vi "calculate phase shift.vi"(6 "dynamically adjust phase?":bool, 9 "integration cluster in":T2={"channel 0"=0, "channel 1"=0, "fly-back heap address"=0, "fly-forward heap address"=0, "xc buffer"=[0, 0, 0, 0, 0]}, 10 "counter cluster in":T3, 11 "scan specification":T1={"x amplitude"=1000, "x resolution (pixels)"=100, "x offset fly-forward (iterations)"=0, "x offset fly-back (iterations)"=0, "y resolution (nr. of lines)"=200, "y step size"=5, "iterations per pixel"=5, "number of frames"=-1, "y offset (pixels)"=0, "number of y-brake lines  (before y-fly-back)"=2, "number y-brake lines (after y-fly-back)"=2, "number of y-fly-back steps"=2, "lines per z step"=5, "number of z/intensity tuples"=200, "number of repetitions (volumes or planes)"=500, "z step size derived"=0, "choose the beginning of z scan"=FALSE, "number of frames (settings)"=0, "FPGA trajectory?"=FALSE}) -> (1 "integration cluster out":T2, 2 "calculated phase shift (iterations)":i16, 3 "scan specification out":T1)   [LabVIEW 2010]
uses:
  counter_cluster.ctl
  integration_cluster.ctl
  scan_specification_cluster.ctl
  <vilib>/rvi/FXPMathLib/FxpMul/XNode/nifxpmath_Multiplier.xnode
  <vilib>/rvi/FXPMathLib/FxpMul/subVIs/nifxpmath_Mul_SimConfig.ctl
  <vilib>/fxp/LVFixedPointQuantizationPolicyTypeDef.ctl
  <vilib>/fxp/LVFixedPointOverflowPolicyTypeDef.ctl
  <vilib>/rvi/FXPMathLib/FxpMul/simVIs/DllFxpMulTemp_sub.vi
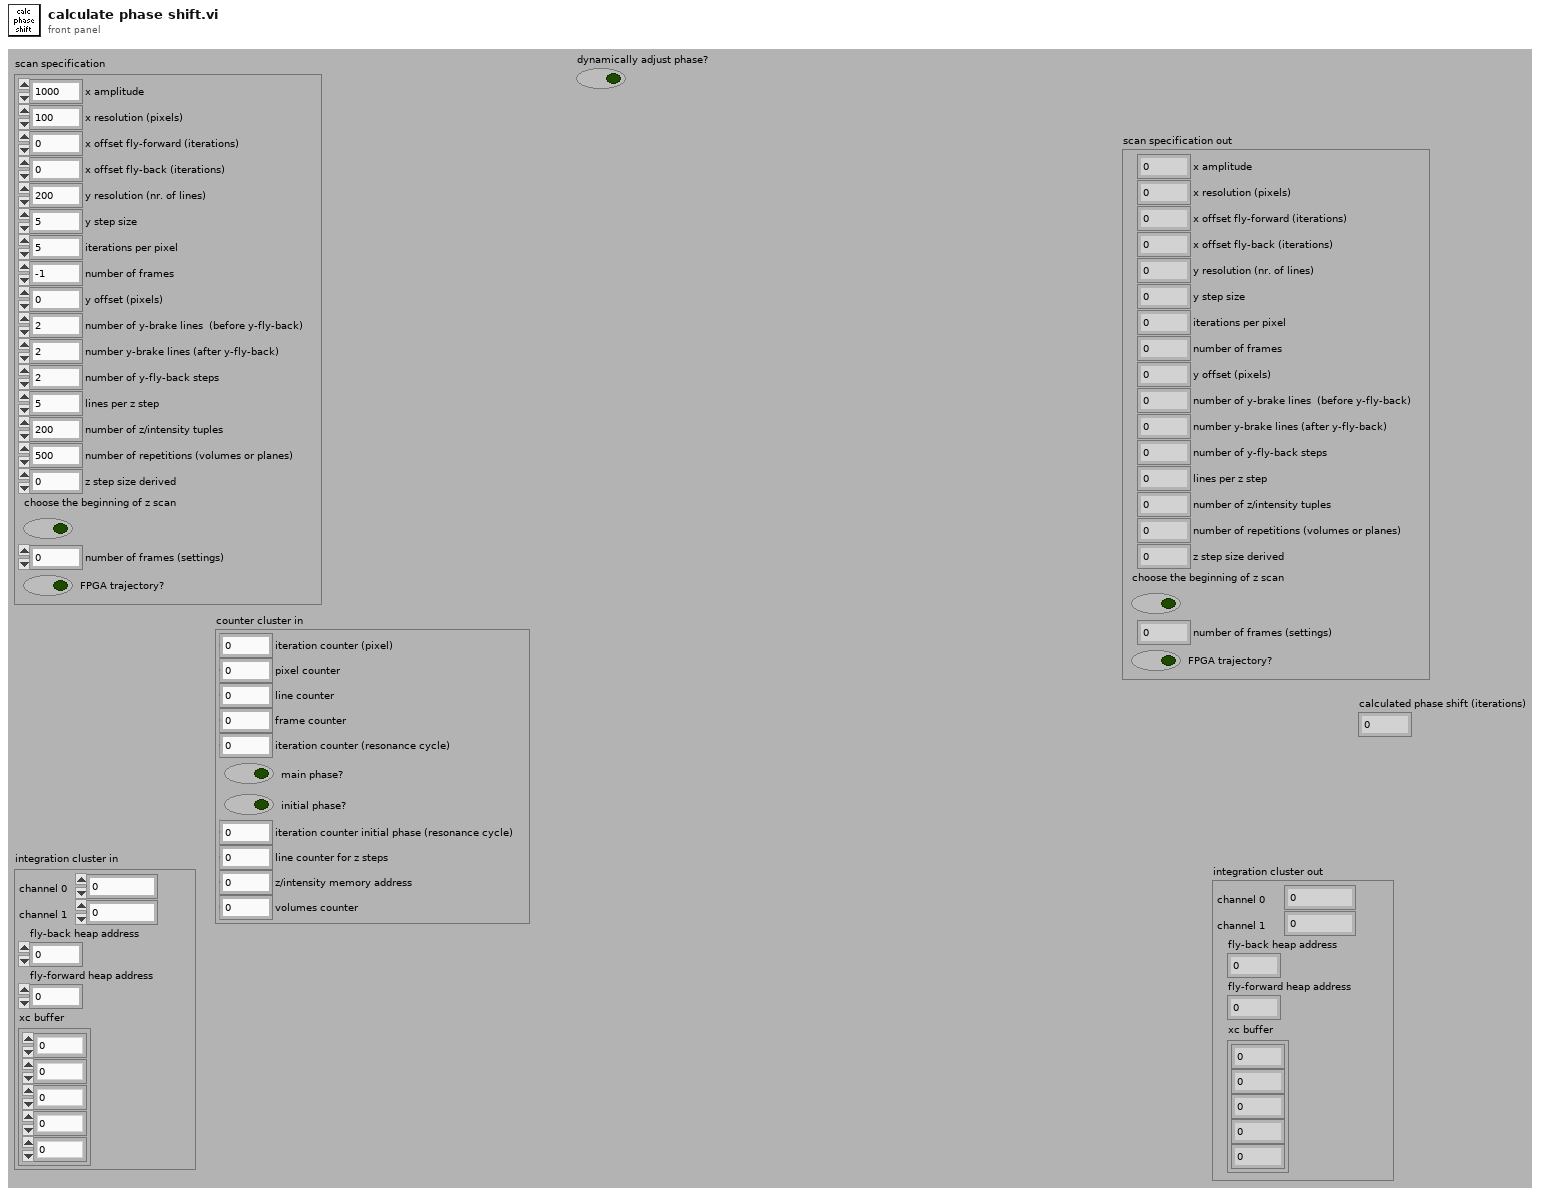
[diagram p1: front panel]
types:
  T1 = typedef "scan_specification_cluster.ctl" = cluster{"x amplitude":u16, "x resolution (pixels)":u16, "x offset fly-forward (iterations)":u16, "x offset fly-back (iterations)":u16, "y resolution (nr. of lines)":u16, "y step size":u16, "iterations per pixel":u16, "number of frames":i32, "y offset (pixels)":u16, "number of y-brake lines  (before y-fly-back)":u16, "number y-brake lines (after y-fly-back)":u16, "number of y-fly-back steps":u16, "lines per z step":u16, "number of z/intensity tuples":u16, "number of repetitions (volumes or planes)":i32, "z step size derived":u16, "choose the beginning of z scan":bool, "number of frames (settings)":i32, "FPGA trajectory?":bool}
  T2 = typedef "integration_cluster.ctl" = cluster{"channel 0":u32, "channel 1":u32, "fly-back heap address":u32, "fly-forward heap address":u32, "xc buffer":u32[]}
  T3 = typedef "counter_cluster.ctl" = cluster{"iteration counter (pixel)":u16, "pixel counter":u16, "line counter":u16, "frame counter":u16, "iteration counter (resonance cycle)":u16, "main phase?":bool, "initial phase?":bool, "iteration counter initial phase (resonance cycle)":u16, "line counter for z steps":u16, "z/intensity memory address":u32, "volumes counter":u16}
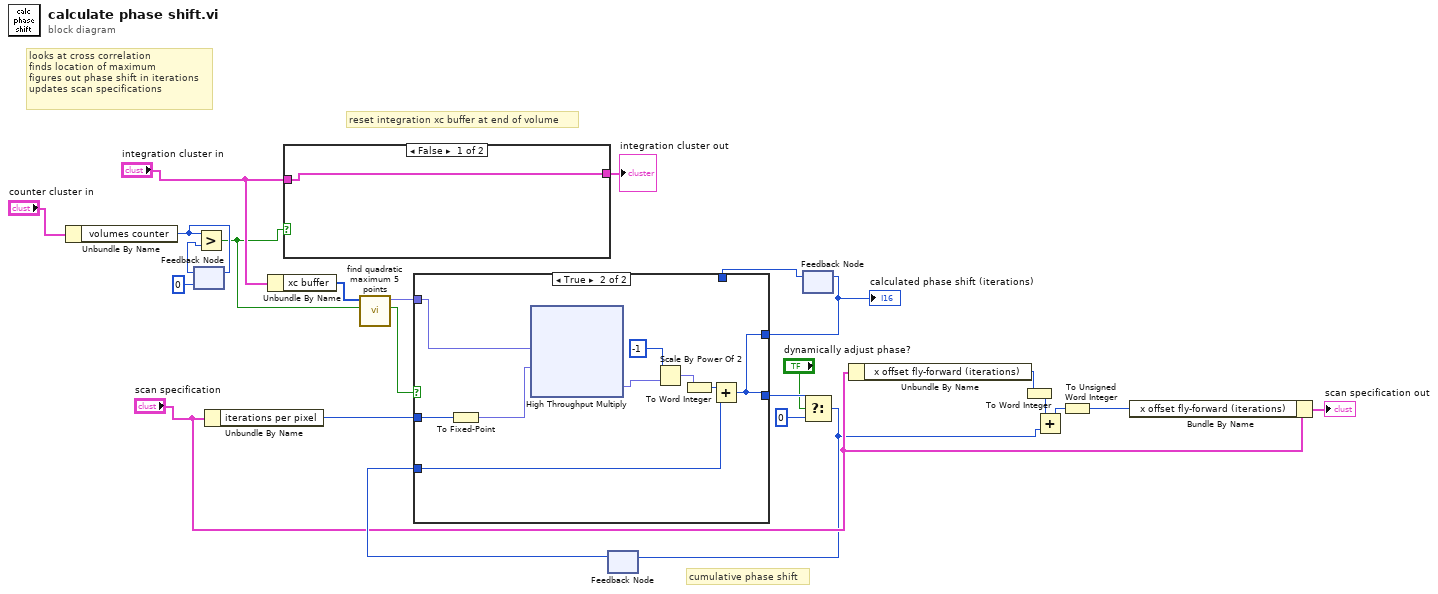
[diagram p0: block diagram]
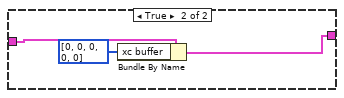
[diagram p3: hidden frame]
diagram:
  # "cumulative phase shift"
  # "reset integration xc buffer at end of volume"
  # "looks at cross correlation\nfinds location of maximum\nfigures out phase shift in iterations\nupdates scan specifications"
  n1 = Unbundle By Name("counter cluster in") -> ("volumes counter"=w22:u16)
  n2 = feedback-in #1(w22) -> ()
  n3 = feedback #1(u16 0 ("volumes counter")) -> (w23:u16)
  n4 = Greater?(x=w22, y=w23) -> (0:w18:bool)
  n5 = Unbundle By Name("scan specification") -> ("iterations per pixel"=w15:u16)
  n6 = Unbundle By Name("integration cluster in") -> ("xc buffer"=w19:u32[])
  n7 = case shown="False" w18 {
    tunnel: "integration cluster in" -> [w25 w28]
    tunnel: [w25 w26] -> w13
    frame False {
    }
    frame True {
      n8 = Bundle By Name(cluster=w28, "xc buffer"=u32[] [0, 0, 0, 0, 0]) -> (w26:T2)
    }
  }
  "integration cluster out" <- w13
  n9 = call "find quadratic maximum 5 points.vi"("input valid"=w18, "xc buffer"=w19) -> ("output valid"=w17:bool, "maximum location"=w16:fxp<+/-,8,3>)  [unwired: 8 in]
  n10 = feedback #2() -> (w14:i16)  [unwired: 1 in]
  n11 = feedback #3() -> (w3:i16)  [unwired: 1 in]
  n12 = case shown="True" w17 {
    tunnel: w16 -> [_ w39]
    tunnel: w15 -> [_ w32]
    tunnel: [w30 w31] -> w12
    tunnel: w14 -> [w30 w37]
    tunnel: [w29 w31] -> w2
    tunnel: w3 -> [w29 _]
    frame False {
    }
    frame True {
      n13 = To Fixed-Point(number=w32) -> (fixed-point=w38:fxp<+,16,16>)  [unwired: 1 in]
      n14 = xnode "High Throughput Multiply"("x"=w39, "y"=w38) -> ("x*y"=w34:fxp<+/-,16,16>)
      n15 = Scale By Power Of 2(n=-1, x=w34) -> (x*2^n=w36:fxp<+/-,16,16>)
      n16 = To Word Integer(number=w36) -> (16bit integer=w33:i16)
      n17 = Add(x=w33, y=w37) -> (x+y=w31:i16)
    }
  }
  "calculated phase shift (iterations)" <- w2
  n18 = feedback-in #3(w2) -> ()
  n19 = Select(t=w12, s="dynamically adjust phase?", f=i16 0) -> (s? t:f=w7:i16)
  n20 = feedback-in #2(w7) -> ()
  n21 = Unbundle By Name("scan specification") -> ("x offset fly-forward (iterations)"=w8:u16)
  n22 = To Word Integer(number=w8) -> (16bit integer=w5:i16)
  n23 = Add(x=w5, y=w7) -> (x+y=w6:i16)
  n24 = To Unsigned Word Integer(number=w6) -> (unsigned 16bit integer=w4:u16)
  n25 = Bundle By Name(cluster="scan specification", "x offset fly-forward (iterations)"=w4) -> (→"scan specification out":T1)
